vi "Global Optimization.vi"(0 "Init Parameters":dbl[][](array[numeric]), 1 "objective and constraint function":refnum<vi>, 2 "function data":variant, 5 "Bounds":cluster{"Min":dbl[], "Max":dbl[]}, 9 "Beginning State":T2, 11 "error in (no error)":errorcluster, 12 "DE settings":T4={"population size"=10, "scale factor"=0.9, "crossover probability"=0.95, "bound mapping method"=1, "mutation method"=0, "crossover method"=0} {"crossover method" items=["Uniform", "Exponential"]; "mutation method" items=["Random", "Either Or", "Best", "Target to Best"]; "bound mapping method" items=["None", "Random between Bounds and Values", "Re-Initialize"]}, 13 "stopping criteria":T1={"max iterations"=50, "max function calls"=-1, "max time (sec)"=-1.0}) -> (3 "number of function calls":i32, 4 "Minimum":dbl[](array[numeric]), 6 "F(Minimum)":dbl[](array[numeric]), 10 "Ending State":T2, 15 "error out":errorcluster)   [LabVIEW 2017, in "NI_AAL_GlobalOptimization.lvlib"]
doc: "Solves a global optimization equation with boundary constraints, nonlinear equality constraints, and nonlinear inequality constraints using the differential evolution (DE) method."
uses:
  <vilib>/gmath/NI_AAL_GlobalOptimization.lvlib
  <vilib>/gmath/GlobalOptimization.llb/DE_Settings.ctl
  <vilib>/gmath/GlobalOptimization.llb/DE_Bound Mapping Method.ctl
  <vilib>/gmath/GlobalOptimization.llb/DE_Mutation Method.ctl
  <vilib>/gmath/GlobalOptimization.llb/DE_Crossover Method.ctl
  <vilib>/gmath/GlobalOptimization.llb/DE_State.ctl
  <vilib>/gmath/GlobalOptimization.llb/DE_Population.ctl
  <vilib>/gmath/GlobalOptimization.llb/DE_Stopping Criteria.ctl
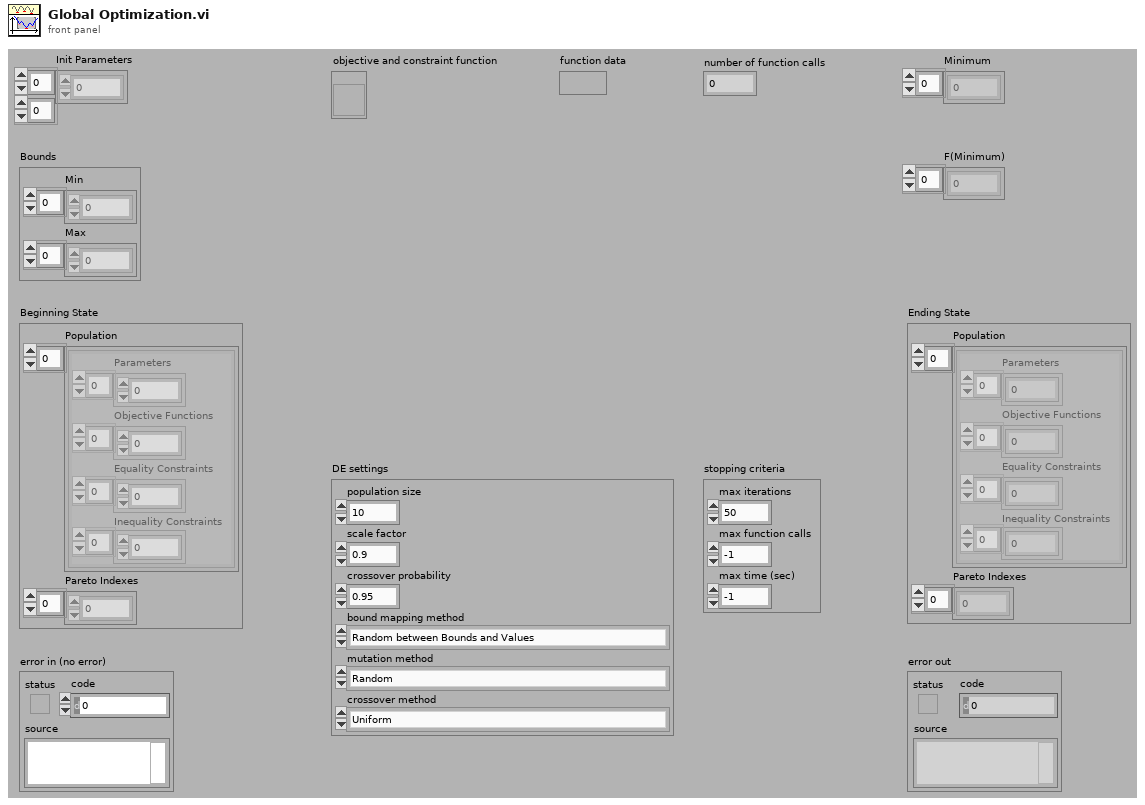
[diagram p1: front panel]
types:
  T1 = typedef "NI_AAL_GlobalOptimization.lvlib/DE_Stopping Criteria.ctl" = cluster{"max iterations":i32, "max function calls":i32, "max time (sec)":dbl}
  T2 = typedef "NI_AAL_GlobalOptimization.lvlib/DE_State.ctl" = cluster{"Population":T3[], "Pareto Indexes":i32[]}
  T3 = typedef "NI_AAL_GlobalOptimization.lvlib/DE_Population.ctl" = cluster{"Parameters":dbl[], "Objective Functions":dbl[], "Equality Constraints":dbl[], "Inequality Constraints":dbl[]}
  T4 = typedef "NI_AAL_GlobalOptimization.lvlib/DE_Settings.ctl" = cluster{"population size":i32, "scale factor":dbl, "crossover probability":dbl, "bound mapping method":T5, "mutation method":T6, "crossover method":T7}
  T5 = typedef "NI_AAL_GlobalOptimization.lvlib/DE_Bound Mapping Method.ctl" = u16
  T6 = typedef "NI_AAL_GlobalOptimization.lvlib/DE_Mutation Method.ctl" = u16
  T7 = typedef "NI_AAL_GlobalOptimization.lvlib/DE_Crossover Method.ctl" = u16
  T8 = typedef "NI_AAL_GlobalOptimization.lvlib/DE_Stopping State.ctl" = cluster{"max iterations":i32, "max function calls":i32, "max time (sec)":dbl, "cur function calls":i32, "init tick count":u32}
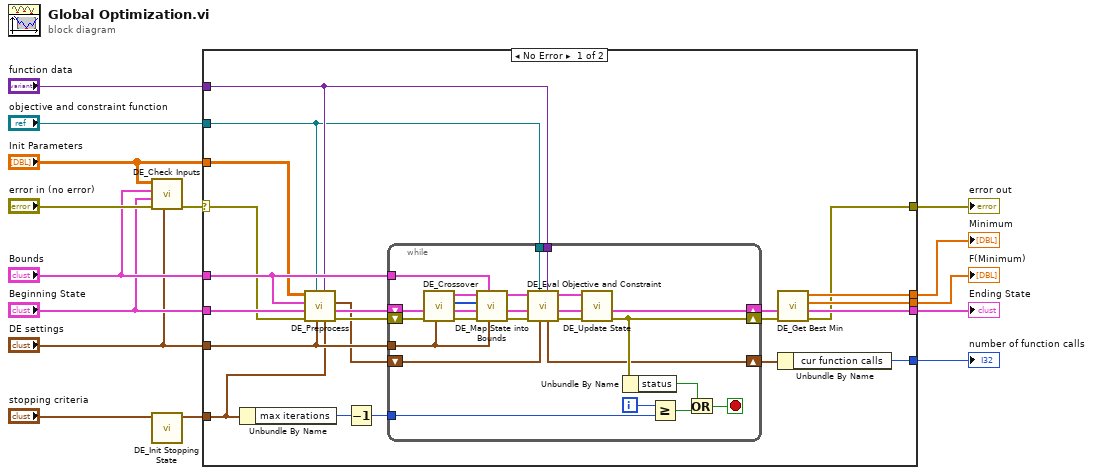
[diagram p0: block diagram]
diagram:
  n1 = call <vilib>:"DE_Check Inputs.vi"("DE settings"="DE settings", "error in (no error)"="error in (no error)", "Beginning State"="Beginning State", "Bounds"="Bounds", "Init Parameters"="Init Parameters") -> ("error out"=w8:errorcluster)  [unwired: 6 in]
  n2 = call <vilib>:"DE_Init Stopping State.vi"("stopping criteria"="stopping criteria") -> ("stopping state"=w1:T8)  [unwired: 10 in]
  n3 = case shown="No Error" w8 {
    selector: w8 -> [w16 w61]
    tunnel: "objective and constraint function" -> [w22 _]
    tunnel: "function data" -> [w25 _]
    tunnel: "DE settings" -> [w28 _]
    tunnel: "Bounds" -> [w29 _]
    tunnel: [w33 _] -> w13
    tunnel: [w32 _] -> w12
    tunnel: [w31 _] -> w11
    tunnel: [w21 w61] -> w10
    tunnel: "Beginning State" -> [w24 _]
    tunnel: [w18 _] -> w9
    tunnel: "Init Parameters" -> [w20 _]
    tunnel: w1 -> [w17 _]
    frame No Error {
      n4 = Unbundle By Name(w17) -> ("max iterations"=w36:i32)
      n5 = call <vilib>:"DE_Preprocess.vi"("stopping state in"=w17, "function data"=w25, "DE settings"=w28, "objective and constraint function"=w22, "error in (no error)"=w16, "State In"=w24, "Bounds"=w29, "Init Parameters"=w20) -> ("error out"=w26:errorcluster, "State Out"=w27:T2, "stopping state out"=w23:T8)  [unwired: 1 in]
      n6 = Decrement(x=w36) -> (x-1=w35:i32)
      n7 = while {
        shift-right: [w55] -> w34
        shift-left: w27 -> [w44]
        shift-right: [w54] -> w30
        shift-left: w26 -> [w43]
        tunnel: w35 -> [w59]
        tunnel: w25 -> [w51]
        shift-right: [w39] -> w19
        shift-left: w23 -> [w40]
        tunnel: w28 -> [w47]
        tunnel: w29 -> [w38]
        tunnel: w22 -> [w41]
        i -> [w60]
        stop <- w56 stop-if-true
        n8 = call <vilib>:"DE_Crossover.vi"("DE settings"=w47, "error in (no error)"=w43, "State In"=w44) -> ("error out"=w45:errorcluster, "State Out"=w46:T2, "Base Indexes"=w37:i32[], "Candidate State"=w42:T2)  [unwired: 5 in]
        n9 = call <vilib>:"DE_Map State into Bounds.vi"("DE settings"=w47, "Bounds"=w38, "error in (no error)"=w45, "State In"=w46, "Base Indexes"=w37, "Candidate State In"=w42) -> ("error out"=w48:errorcluster, "State Out"=w49:T2, "Candidate State Out"=w50:T2)  [unwired: 3 in]
        n10 = call <vilib>:"DE_Eval Objective and Constraint.vi"("function data"=w51, "stopping state in"=w40, "objective and constraint function"=w41, "error in (no error)"=w48, "State In"=w50) -> ("error out"=w53:errorcluster, "State Out"=w52:T2, "stopping state out"=w39:T8)  [unwired: 4 in]
        n11 = call <vilib>:"DE_Update State.vi"("error in (no error)"=w53, "State In"=w49, "Candidate State"=w52) -> ("error out"=w54:errorcluster, "State Out"=w55:T2)  [unwired: 7 in]
        n12 = Unbundle By Name(w54) -> ("status"=w58:bool)
        n13 = Greater Or Equal?(x=w60, y=w59) -> (x >= y?=w57:bool)
        n14 = Or(x=w58, y=w57) -> (x .or. y?=w56:bool)
      }
      n15 = call <vilib>:"DE_Get Best Min.vi"("error in (no error)"=w30, "State In"=w34) -> ("error out"=w21:errorcluster, "State Out"=w33:T2, "F(Minimum)"=w31:dbl[], "Minimum"=w32:dbl[])  [unwired: 6 in]
      n16 = Unbundle By Name(w19) -> ("cur function calls"=w18:i32)
    }
    frame Error {
    }
  }
  "Minimum" <- w12
  "F(Minimum)" <- w11
  "error out" <- w10
  "Ending State" <- w13
  "number of function calls" <- w9
